vi "Unflatten JSONpath Array to Object.vi"(8 "error in (no error)":errorcluster, 9 "JSON Items":string[](array[string]), 10 "Initial JSON Object":string="{}", 11 "$Paths":string[](array[string])) -> (0 "error out":errorcluster, 3 "<JSON>":string)   [LabVIEW 2020, in "JSONtext.lvlib"]
doc: "Takes arrays of $Paths items and generates a Object containing those $Paths. Does not support multi-point paths.\n\nFor example: the $Paths (Items):\n$.A.B1 (1)\n$.A.B2 (\"x\")\n$.A2 (true)\n$.A3.C (123)\nproduce the JSON: {\"A\":{\"B1\":1\"B2:\"x\"},\"A2\":true,\"A3\":{\"C\":123}}"
uses:
  <vilib>/JDP Science/JSONtext/JSONtext.lvlib
  <vilib>/JDP Science/JSONtext/Parsing/Advance past whitespace.vi
  <vilib>/JDP Science/JSONtext/Parsing/Match Pattern.vi
  <vilib>/JDP Science/JSONtext/support/Quote and Escape JSON string.vi
  <vilib>/JDP Science/JSONtext/Parsing/Advance past String.vi
  <vilib>/JDP Science/JSONtext/String Subset.vi
  <vilib>/JDP Science/JSONtext/Parsing/Advance past whitespace and comma.vi
  <vilib>/JDP Science/JDP Science Common Utilities/Trim Whitespace__JDP.vi
  <vilib>/JDP Science/JSONtext/Parsing/Replace at Offset.vi
  <vilib>/JDP Science/JSONtext/support/Make empty strings null.vi
  <vilib>/JDP Science/JSONtext/Parsing/Advance past Line Ending.vi
  <vilib>/JDP Science/JSONtext/support/quote and escape json string 2.vi
  <vilib>/JDP Science/JSONtext/Parsing/Advance past replacable whitespace.vi
  <vilib>/JDP Science/JSONtext/Parsing/Parsing Error.vi
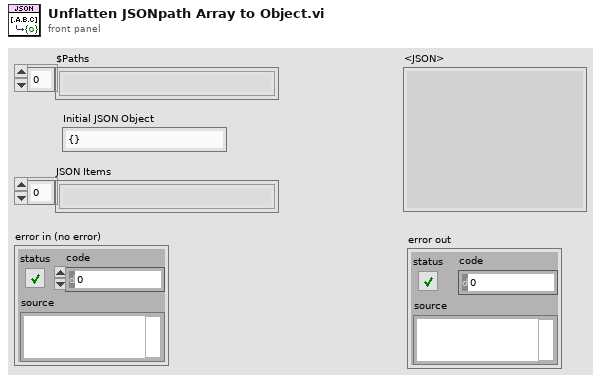
[diagram p1: front panel]
types:
  T1 = typedef "JSONtext.lvlib/Found Items.ctl" = cluster{"Item offset":i32, "Offset past Item":i32, "Name offset":i32, "Offset past Name":i32, "Found":bool, "Item Type":T2, "Item Index":i32, "Start Offset":i32, "Comma Needed For Insert":T3}
  T2 = typedef "JSONtext.lvlib/Parsing State.ctl" = enum16{"Parser Error", "Object", "Array", "String", "Number/Other", "Leading Whitespace", "Object end", "Array end", "Value end"}
  T3 = typedef "JSONtext.lvlib/Comma Needed for Insert.ctl" = enum8{"False", "True", "Following"}
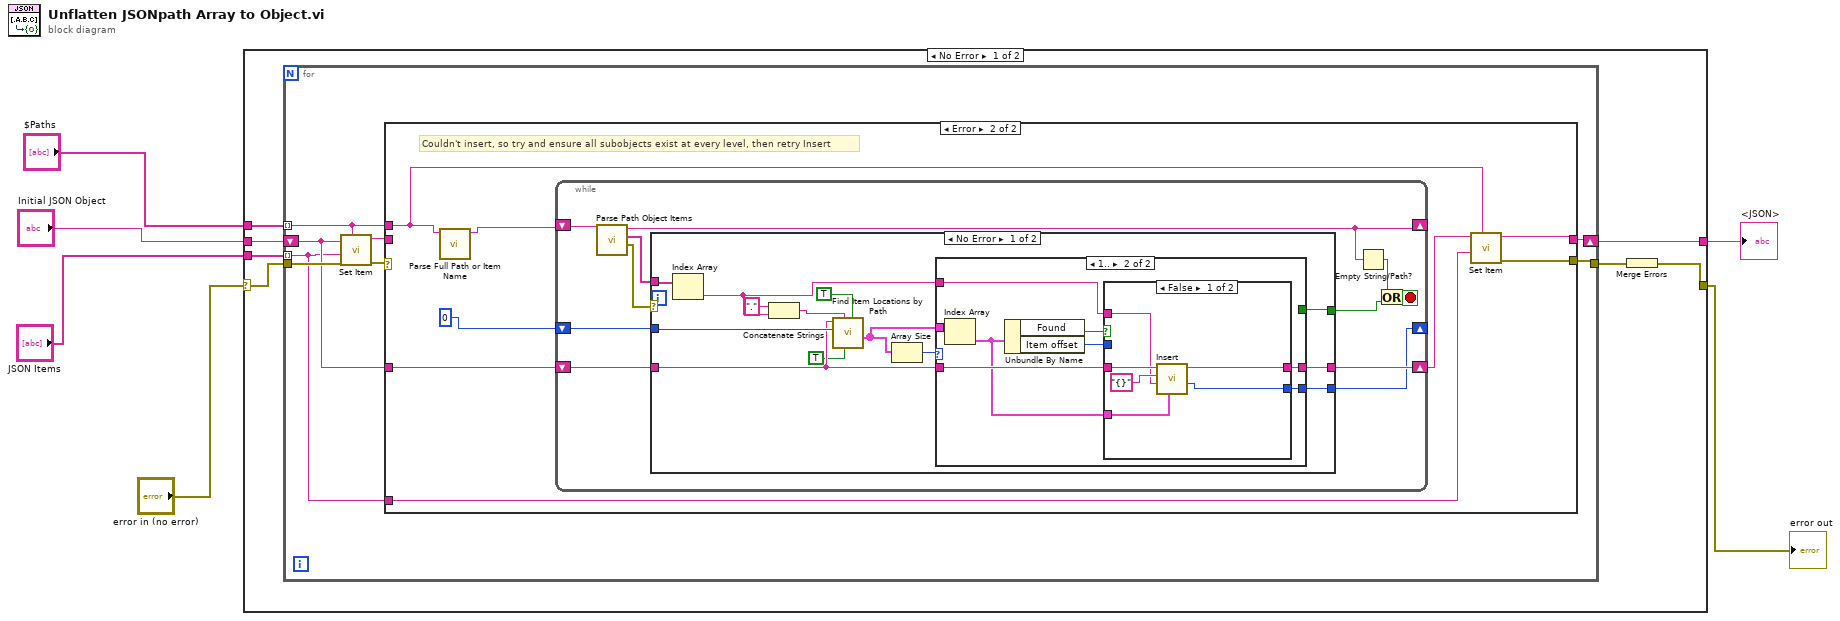
[diagram p0: block diagram]
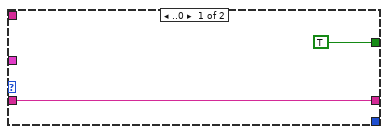
[diagram p3: hidden frame]
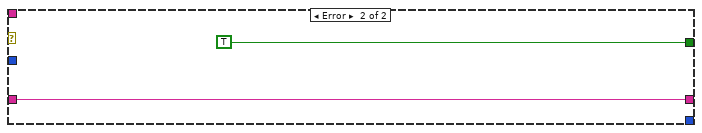
[diagram p5: hidden frame]
diagram:
  n1 = case shown="No Error" "error in (no error)" {
    selector: "error in (no error)" -> [w11 w76]
    tunnel: "$Paths" -> [w13 _]
    tunnel: "JSON Items" -> [w12 _]
    tunnel: [w10 _] -> w5
    tunnel: [w8 w76] -> w6
    tunnel: "Initial JSON Object" -> [w7 _]
    frame No Error {
      n2 = for {
        tunnel: w13 -> [w19] mode=indexing
        shift-right: [w16] -> w10
        shift-left: w7 -> [w18]
        tunnel: w12 -> [w14] mode=indexing
        tunnel: w11 -> [w21]
        tunnel: [w15] -> w9
        n3 = call <vilib>:"Set Item.vi"("$Path or Item Name"=w19, "error in (no error)"=w21, "JSON to Insert"=w14, "JSON"=w18) -> ("error out"=w20:errorcluster, "<JSON>"=w17:string)  [unwired: 4 in, 1 out]
        n4 = case shown="Error" w20 {
          selector: w20 -> [w22 _]
          tunnel: w19 -> [_ w26]
          tunnel: w18 -> [_ w31]
          tunnel: w17 -> [w23 _]
          tunnel: [w23 w29] -> w16
          tunnel: [w22 w28] -> w15
          tunnel: w14 -> [_ w27]
          frame No Error {
          }
          frame Error {
            # "Couldn't insert, so try and ensure all subobjects exist at every level, then retry Insert"
            n5 = call <vilib>:"Parse Full Path or Item Name.vi"("Full Path (with $) or Name"=w26) -> ("Relative Path or JSON-format name"=w24:string)  [unwired: 10 in]
            n6 = while {
              shift-right: [w40] -> _
              shift-left: w24 -> [w34]
              shift-right: [w37] -> w30
              shift-left: w31 -> [w38]
              shift-right: [w32] -> _
              shift-left: 0 ("Offset") -> [w33]
              stop <- w36 stop-if-true
              n7 = call <vilib>:"Parse Path Object Items.vi"("Path with leading Object element"=w34) -> ("error out"=w41:errorcluster, "<JSON>items names"=w39:string[], "Rest or Path"=w40:string)  [unwired: 7 in, 1 out]
              n8 = case shown="No Error" w41 {
                tunnel: w39 -> [w55 _]
                tunnel: w38 -> [w52 w74]
                tunnel: [w54 w74] -> w37
                tunnel: [w44 TRUE] -> w35
                tunnel: w33 -> [w53 _]
                tunnel: [w49 _] -> w32
                frame No Error {
                  n9 = Index Array(array=w55) -> (element=w47:string)  [unwired: 1 in]
                  n10 = Concatenate Strings("." ("string"), w47) -> (w48:string)
                  n11 = call <vilib>:"Find Item Locations by Path.vi"("Insertion point if not found"=TRUE, "Only return first found"=TRUE, "Path"=w48, "Offset"=w53, "JSON"=w52) -> ("Items"=w46:T1[])  [unwired: 5 in, 1 out]
                  n12 = Array Size(array=w46) -> (size(s)=w45:i32)
                  n13 = case shown="1.." w45 {
                    tunnel: [w57 w65] -> w54
                    tunnel: w52 -> [w57 w64]
                    tunnel: [_ w61] -> w49
                    tunnel: w47 -> [_ w59]
                    tunnel: w46 -> [_ w58]
                    tunnel: [TRUE _] -> w44
                    frame ..0 {
                    }
                    frame 1.. {
                      n14 = Index Array(array=w58) -> (element=w62:T1)  [unwired: 1 in]
                      n15 = Unbundle By Name(w62) -> ("Found"=w63:bool, "Item offset"=w60:i32)
                      n16 = case shown="False" w63 {
                        tunnel: [w69 w73] -> w65
                        tunnel: w64 -> [w70 w73]
                        tunnel: w62 -> [w71 _]
                        tunnel: w59 -> [w67 _]
                        tunnel: [w66 w72] -> w61
                        tunnel: w60 -> [_ w72]
                        frame False {
                          n17 = call <vilib>:"Insert.vi"("Item"=w71, "<JSON>name"=w67, "JSON to Insert"="{}", "JSON in"=w70) -> ("Inserted Item Offset"=w66:i32, "string"=w69:string)  [unwired: 5 in, 1 out]
                        }
                        frame True {
                        }
                      }
                    }
                  }
                }
                frame Error {
                }
              }
              n18 = Empty String/Path?(string/path=w40) -> (empty?=w42:bool)
              n19 = Or(x=w42, y=w35) -> (x .or. y?=w36:bool)
            }
            n20 = call <vilib>:"Set Item.vi"("$Path or Item Name"=w26, "JSON to Insert"=w27, "JSON"=w30) -> ("error out"=w28:errorcluster, "<JSON>"=w29:string)  [unwired: 5 in, 1 out]
          }
        }
      }
      n21 = Merge Errors(w9) -> (w8:errorcluster)
    }
    frame Error {
    }
  }
  "error out" <- w6
  "<JSON>" <- w5
